vi "DriveMotorTest.vi"() -> ()   [LabVIEW 2015]
uses:
  Support/Global Objects.vi
panel:
  in  "Output":dbl
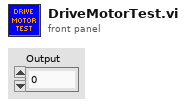
[diagram p1: front panel]
types:
  T1 = typedef "2 Motor Typedef.ctl" = cluster{"Motor1":T2, "Motor2":T2, "Last Motor Power":dbl}
  T2 = typedef "WPI_MotorControlDeviceRef.ctl" = cluster{"DeviceStatus":errorcluster, "Type":T3, "PWM":cluster{"PWM Channel":T4, "DeadBand":T5}, "CAN":cluster{"Device Number":u8, "Control Mode":T6, "Semaphore":T7, "Max Vout":dbl, "TalonSRX Control Mode":T8}, "Invert":bool}
  T3 = typedef "WPI_MotorControlType.ctl" = enum16{"PWM", "CAN", "CANTalonSRX"}
  T4 = typedef "FPGA_DIOPWMChannel.ctl" = enum8{"PWM 0", "PWM 1", "PWM 2", "PWM 3", "PWM 4", "PWM 5", "PWM 6", "PWM 7", "PWM 8", "PWM 9", "PWM MXP 0", "PWM MXP 1", "PWM MXP 2", "PWM MXP 3", "PWM MXP 4", "PWM MXP 5", "PWM MXP 6", "PWM MXP 7", "PWM MXP 8", "PWM MXP 9", "Invalid"}
  T5 = typedef "WPI_PWMDeadband.ctl" = cluster{"Name":string, "maxPositivePwm":i32, "minPositivePwm":i32, "centerPwm":i32, "maxNegativePwm":i32, "minNegativePwm":i32, "angularRange":u16}
  T6 = typedef "WPI_CANJaguar_ControlMode.ctl" = enum8{"Percent VBus", "Current", "Speed", "Position", "Voltage"}
  T7 = typedef "Semaphore RefNum" = refnum<k1>
  T8 = typedef "WPI_CANTalonSRX_APIControlMode.ctl" = enum8{"Percent VBus", "Speed", "Position", "Slave", "Unchanged / Invalid", "Voltage Compensation", "Current", "Motion Profile"}
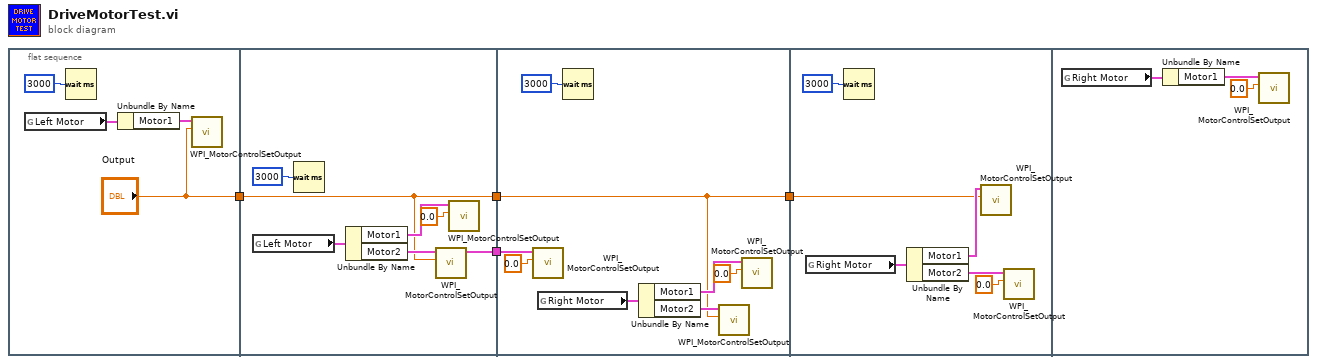
[diagram p0: block diagram]
diagram:
  n1 = flat-sequence {
    tunnel: ["Output"] -> w4
    tunnel: w4 -> [w10]
    tunnel: [w10] -> w3
    tunnel: [w9] -> w2
    tunnel: w3 -> [w16]
    tunnel: w2 -> [w18]
    tunnel: [w16] -> w1
    tunnel: w1 -> [w25]
    frame #0 {
      n2 = global read "Global Objects.vi" "Left Motor"() -> (w8:T1)
      n3 = Wait (ms)(milliseconds to wait=u32 3000) -> ()  [unwired: 1 out]
      n4 = Unbundle By Name(w8) -> ("Motor1"=w7:T2)
      n5 = call <vilib>:"WPI_MotorControlSetOutput.vi"("Output"="Output", "MotorControlDevRef"=w7) -> ()  [unwired: 7 in, 3 out]
    }
    frame #1 {
      n6 = global read "Global Objects.vi" "Left Motor"() -> (w13:T1)
      n7 = Wait (ms)(milliseconds to wait=u32 3000) -> ()  [unwired: 1 out]
      n8 = Unbundle By Name(w13) -> ("Motor1"=w14:T2, "Motor2"=w11:T2)
      n9 = call <vilib>:"WPI_MotorControlSetOutput.vi"("Output"=w10, "MotorControlDevRef"=w11) -> ("MotorControlDevRef"=w9:T2)  [unwired: 7 in, 2 out]
      n10 = call <vilib>:"WPI_MotorControlSetOutput.vi"("Output"=0.0, "MotorControlDevRef"=w14) -> ()  [unwired: 7 in, 3 out]
    }
    frame #2 {
      n11 = call <vilib>:"WPI_MotorControlSetOutput.vi"("Output"=0.0, "MotorControlDevRef"=w18) -> ()  [unwired: 7 in, 3 out]
      n12 = global read "Global Objects.vi" "Right Motor"() -> (w21:T1)
      n13 = Wait (ms)(milliseconds to wait=u32 3000) -> ()  [unwired: 1 out]
      n14 = Unbundle By Name(w21) -> ("Motor1"=w20:T2, "Motor2"=w23:T2)
      n15 = call <vilib>:"WPI_MotorControlSetOutput.vi"("Output"=w16, "MotorControlDevRef"=w23) -> ()  [unwired: 7 in, 3 out]
      n16 = call <vilib>:"WPI_MotorControlSetOutput.vi"("Output"=0.0, "MotorControlDevRef"=w20) -> ()  [unwired: 7 in, 3 out]
    }
    frame #3 {
      n17 = global read "Global Objects.vi" "Right Motor"() -> (w27:T1)
      n18 = Wait (ms)(milliseconds to wait=u32 3000) -> ()  [unwired: 1 out]
      n19 = Unbundle By Name(w27) -> ("Motor1"=w28:T2, "Motor2"=w26:T2)
      n20 = call <vilib>:"WPI_MotorControlSetOutput.vi"("Output"=w25, "MotorControlDevRef"=w28) -> ()  [unwired: 7 in, 3 out]
      n21 = call <vilib>:"WPI_MotorControlSetOutput.vi"("Output"=0.0, "MotorControlDevRef"=w26) -> ()  [unwired: 7 in, 3 out]
    }
    frame #4 {
      n22 = global read "Global Objects.vi" "Right Motor"() -> (w30:T1)
      n23 = Unbundle By Name(w30) -> ("Motor1"=w31:T2)
      n24 = call <vilib>:"WPI_MotorControlSetOutput.vi"("Output"=0.0, "MotorControlDevRef"=w31) -> ()  [unwired: 7 in, 3 out]
    }
  }
